vi "stage_comp_y.vi"(11 "xpos":dbl=53.07 format="%#_13g") -> (2 "zcorr":dbl, 3 "ycorr":dbl)   [LabVIEW 2018]
panel:
  in  "p4y":dbl=53.07 format="%#_13g"
  in  "p3y":dbl=-0.07201 format="%#_13g"
  in  "p2y":dbl=1.86e-05 format="%#_13g"
  in  "p1y":dbl=-5.2e-10 format="%#_13g"
  in  "p4z":dbl=13.76 format="%#_13g"
  in  "p3z":dbl=-0.033 format="%#_13g"
  in  "p2z":dbl=1.324e-05 format="%#_13g"
  in  "p1z":dbl=-2.675e-10 format="%#_13g"
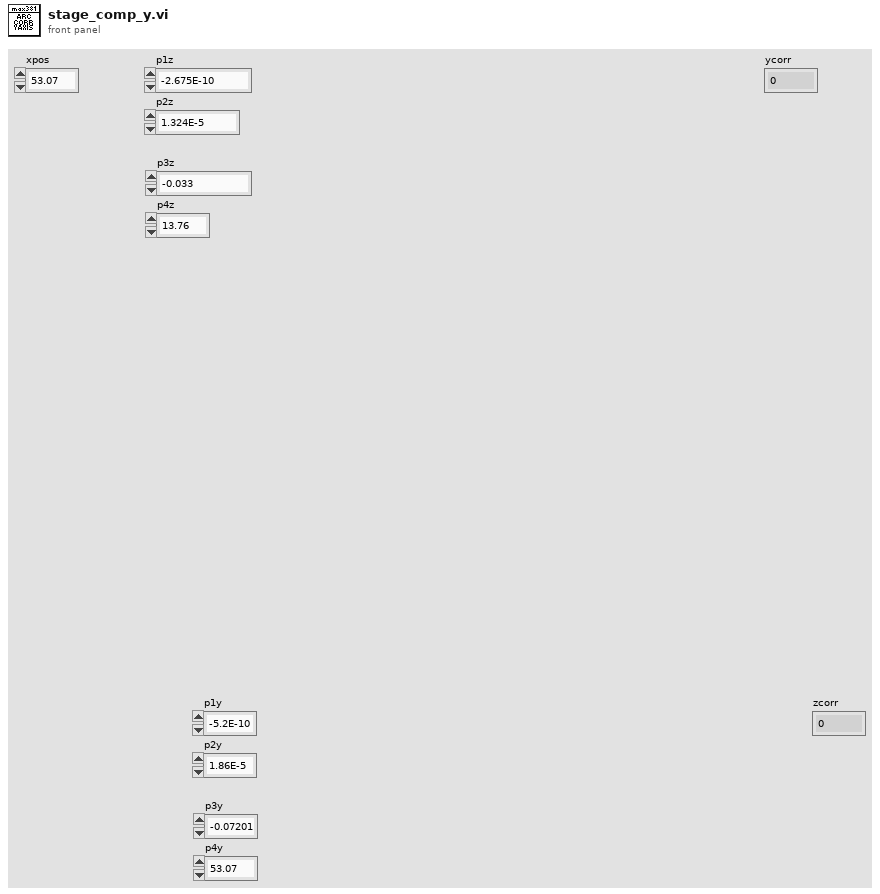
[diagram p1: front panel]
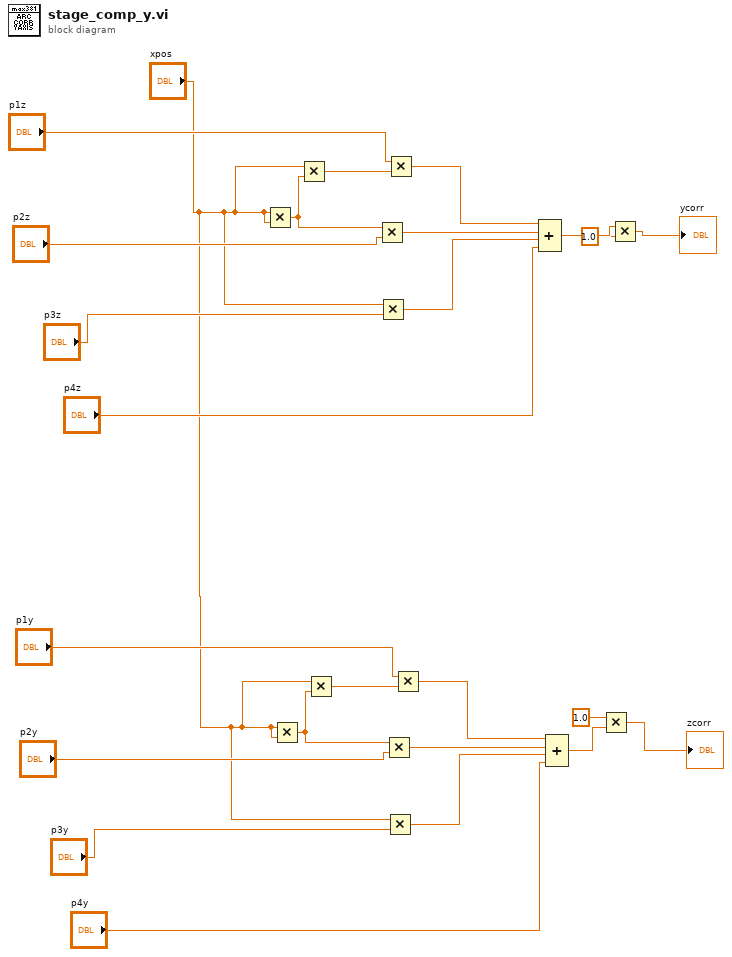
[diagram p0: block diagram]
diagram:
  n1 = Multiply(x="xpos", y="xpos") -> (x*y=w19:dbl)
  n2 = Multiply(x="xpos", y="xpos") -> (x*y=w7:dbl)
  n3 = Multiply(x="xpos", y=w19) -> (x*y=w25:dbl)
  n4 = Multiply(x="xpos", y=w7) -> (x*y=w13:dbl)
  n5 = Multiply(x=w19, y="p2z") -> (x*y=w23:dbl)
  n6 = Multiply(x="xpos", y="p3z") -> (x*y=w22:dbl)
  n7 = Multiply(x=w7, y="p2y") -> (x*y=w11:dbl)
  n8 = Multiply(x="xpos", y="p3y") -> (x*y=w10:dbl)
  n9 = Multiply(x="p1z", y=w25) -> (x*y=w24:dbl)
  n10 = Multiply(x="p1y", y=w13) -> (x*y=w12:dbl)
  n11 = Compound Arithmetic op=ADD(w24, w23, w22, "p4z") -> (w16:dbl)
  n12 = Compound Arithmetic op=ADD(w12, w11, w10, "p4y") -> (w3:dbl)
  n13 = Multiply(x=1.0, y=w3) -> (x*y=→"zcorr":dbl)
  n14 = Multiply(x=w16, y=1.0) -> (x*y=→"ycorr":dbl)
